vi "calcDist.vi"() -> ()   [LabVIEW 2009]
panel:
  out "x*y":dbl
  out "x/y":dbl
  out "x+y":dbl
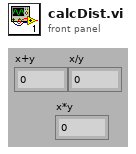
[diagram p1: front panel]
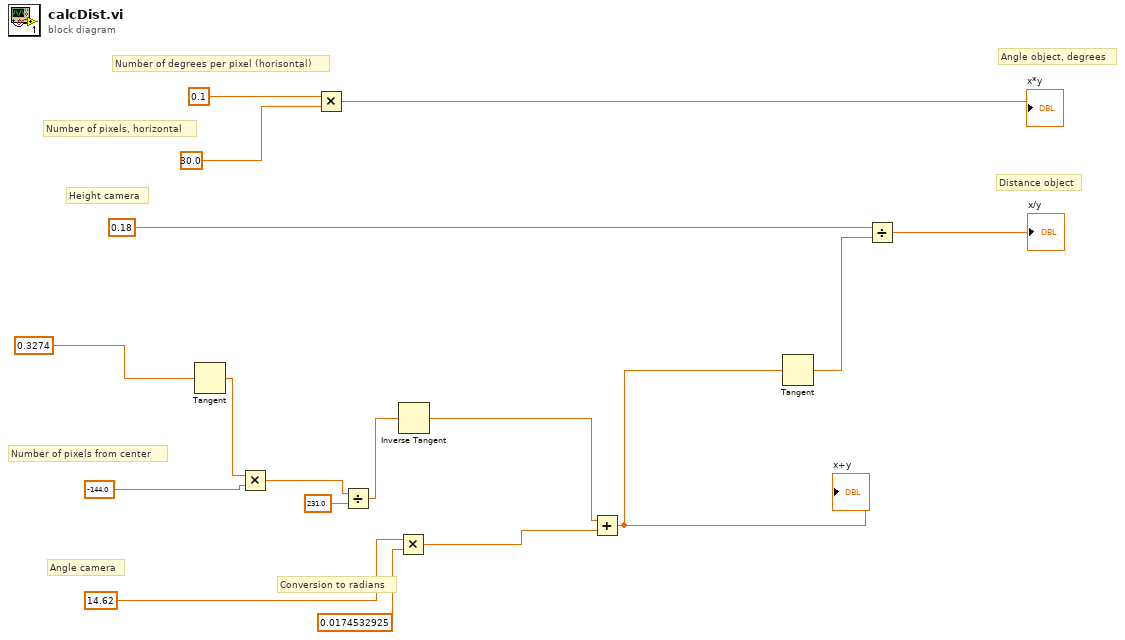
[diagram p0: block diagram]
diagram:
  # "Angle object, degrees"
  # "Number of pixels, horizontal"
  # "Number of degrees per pixel (horisontal)"
  # "Distance object"
  # "Conversion to radians"
  # "Angle camera"
  # "Number of pixels from center"
  # "Height camera"
  n1 = Tangent(1:0.3274 ("x")) -> (0:w8:dbl)
  n2 = Multiply(x=w8, y=-144.0) -> (x*y=w7:dbl)
  n3 = Multiply(x=0.1, y=30.0) -> (x*y=→"x*y":dbl)
  n4 = Divide(x=w7, y=231.0) -> (x/y=w5:dbl)
  n5 = Multiply(x=14.62 ("y"), y=0.0174532925) -> (x*y=w3:dbl)
  n6 = Inverse Tangent(1:w5) -> (0:w2:dbl)
  n7 = Add(x=w2, y=w3) -> (x+y=w1:dbl)
  "x+y" <- w1
  n8 = Tangent(1:w1) -> (0:w14:dbl)
  n9 = Divide(x=0.18, y=w14) -> (x/y=→"x/y":dbl)
